vi "Publish (async,private).vi"(4 "ArgumentsKw":string, 6 "Arguments":string, 7 "Options":string, 8 "Error in":errorcluster, 9 "Request Ack.":bool, 10 "Topic":string, 11 "WAMP Client in":refnum<class "WAMP Client.lvclass">) -> (0 "Error cout":errorcluster, 2 "notifier out":refnum<notifier>, 3 "WAMP Client out":refnum<class "WAMP Client.lvclass">)   [LabVIEW 2020, in "wamplv.lvlib" / "WAMP Client.lvclass"]
uses:
  WAMP Client.lvclass
  TypeDef/PUBLISH result.ctl
  API/TypeDefs/Combined error.ctl
  API/TypeDefs/WAMP error.ctl
  TypeDef/Internal Message Type.ctl
  TypeDef/PUBLISH Request Data.ctl
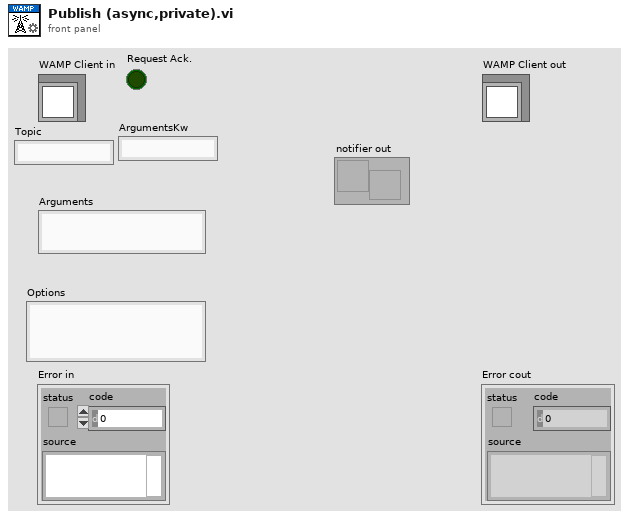
[diagram p1: front panel]
types:
  T1 = typedef "wamplv.lvlib/WAMP Client.lvclass/PUBLISH result.ctl" = cluster{"Publication ID":u64, "Success?":bool, "Combined Error":T2}
  T2 = typedef "wamplv.lvlib/WAMP Client.lvclass/Combined error.ctl" = cluster{"Error?":bool, "WAMP Error":T3, "Error":errorcluster}
  T3 = typedef "wamplv.lvlib/WAMP Client.lvclass/WAMP error.ctl" = cluster{"Details":string, "ArgumentKw Payload":string, "Error?":bool, "Error URI":string, "Arguments Payload":string}
  T4 = typedef "wamplv.lvlib/WAMP Client.lvclass/PUBLISH Request Data.ctl" = cluster{"Topic URI":string, "Arguments":string, "ArgumentsKw":string, "Request Acknowledgement":bool, "Options":string, "Publish result notifier":refnum<notifier>}
  T5 = typedef "wamplv.lvlib/WAMP Client.lvclass/Internal Message Type.ctl" = enum16{"Subscribe", "Handle Subscribed", "Handle Event", "Unsubscribe", "Handle Unsubscribed", "Publish", "Handled Published", "Goodbye", "Handle Goodbye", "Call", "Handle Result", "Register", "Handle Registered", "Unregister", "Handle Unregistered", "Handle Invocation", "Yield", "Error"}
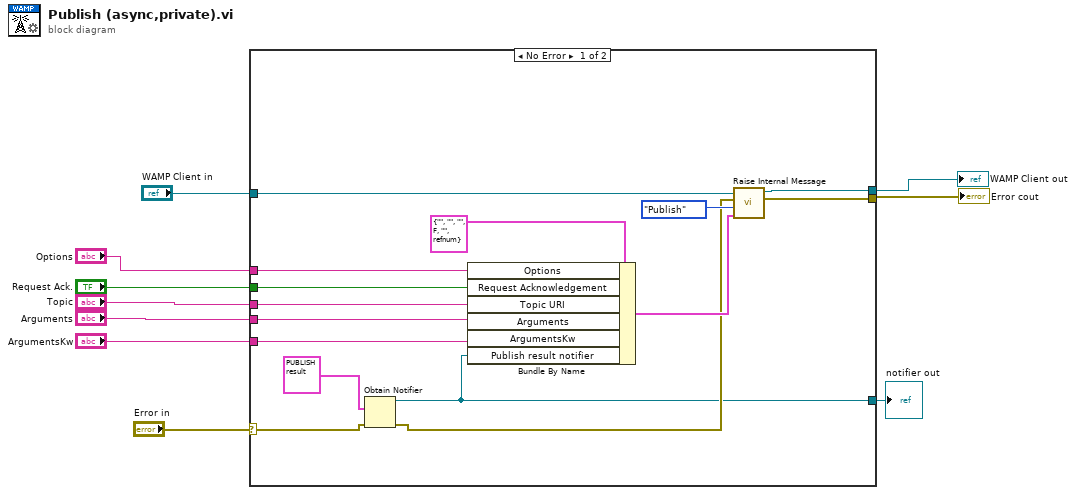
[diagram p0: block diagram]
diagram:
  n1 = case shown="No Error" "Error in" {
    selector: "Error in" -> [w13 w27]
    tunnel: [w20 w27] -> w9
    tunnel: [w19 w26] -> w7
    tunnel: "WAMP Client in" -> [w25 w26]
    tunnel: "Topic" -> [w23 _]
    tunnel: "Arguments" -> [w18 _]
    tunnel: "ArgumentsKw" -> [w17 _]
    tunnel: "Request Ack." -> [w16 _]
    tunnel: "Options" -> [w15 _]
    tunnel: [w12 _] -> w1
    frame No Error {
      n2 = Obtain Notifier(notification data type=T1 {"Publication ID"=0, "Success?"=FALSE, "Combined Error"={"Error?"=FALSE, "WAMP Error"={"Details"="", "ArgumentKw Payload"="{}", "Error?"=FALSE, "Error URI"="", "Arguments Payload"=""}, "Error"={"status"=FALSE, "code"=0, "source"=""}}} ("Cluster"), error in (no error)=w13) -> (notifier out=w12:refnum<notifier>, error out=w14:errorcluster)  [unwired: 2 in, 1 out]
      n3 = Bundle By Name(cluster=T4 {"Topic URI"="", "Arguments"="", "ArgumentsKw"="", "Request Acknowledgement"=FALSE, "Options"="", "Publish result notifier"=refnum} ("Cluster"), "Options"=w15, "Request Acknowledgement"=w16, "Topic URI"=w23, "Arguments"=w18, "ArgumentsKw"=w17, "Publish result notifier"=w12) -> (w24:T4)
      n4 = call-dynamic "Raise Internal Message.vi"("Variant"=w24, "Internal Message Type"=Internal_Message_Type."Publish", "error in (no error)"=w14, "WAMP Client in"=w25) -> ("error out"=w20:errorcluster, "WAMP Client out"=w19:refnum<class "WAMP Client.lvclass">)  [unwired: 6 in]
    }
    frame Error {
    }
  }
  "Error cout" <- w9
  "WAMP Client out" <- w7
  "notifier out" <- w1
